vi "Blinking_Led_13.vi"() -> ()   [LabVIEW 2018]
uses:
  <vilib>/MakerHub/LINX/Public/Peripherals/Digital/Digital Write 1 Chan.vi
  <vilib>/MakerHub/LINX/Public/Peripherals/Digital/Digital Write N Chans.vi
  <vilib>/MakerHub/LINX/Private/Local IO/LinxDigitalWrite.vi
  <vilib>/MakerHub/LINX/Public/Utilities/Check Channel.vi
  <vilib>/MakerHub/LINX/Public/Utilities/Open Serial.vi
  <vilib>/MakerHub/LINX/Private/Utilties/Generate Error.vi
  <vilib>/MakerHub/LINX/LMH-LINX.lvlib
panel:
  in  "milliseconds Toff":u32=500
  in  "milliseconds Ton":u32=500
  in  "Repeticiones blink":i32=6
  in  "DO Channel":u8=13 min=2 step=1
  in  "Serial Port":refnum<visa-resource-name>="COM3"
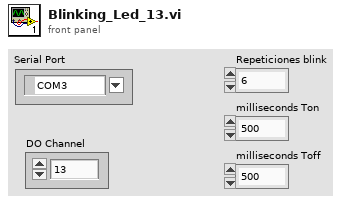
[diagram p1: front panel]
types:
  T1 = typedef "LMH-LINX.lvlib/LINX Ref.ctl" = cluster{"IO":T2, "Interface":T3, "LINX Device Config":T4}
  T2 = typedef "LMH-LINX.lvlib/Platform.ctl" = enum16{"Remote", "Local"}
  T3 = typedef "LMH-LINX.lvlib/Interface.ctl" = enum16{"Serial", "TCP"}
  T4 = typedef "LMH-LINX.lvlib/Device.lvlib/LINX Device Config.ctl" = cluster{"Interface":T3, "COM Port":refnum<visa-resource-name>, "TCP Configuration":T5, "Device Family":u8, "Device ID":u8, "Device Name":string, "TCP Ref":refnum<k5>, "Channels":T6}
  T5 = typedef "LMH-LINX.lvlib/Device.lvlib/TCP Config.ctl" = cluster{"IP Address":string, "Port":u16}
  T6 = typedef "LMH-LINX.lvlib/Channels.ctl" = cluster{"DI":u8[], "DO":u8[], "AI":u8[], "AO":u8[], "PWM":u8[], "QE":u8[], "UART":u8[], "I2C 2":u8[], "SPI":u8[], "CAN":u8[], "Servo":u8[], "AI Ref (V)":dbl, "AI Resolution (Bits)":u8, "AO Ref (V)":dbl, "AO Resolution (Bits)":u8}
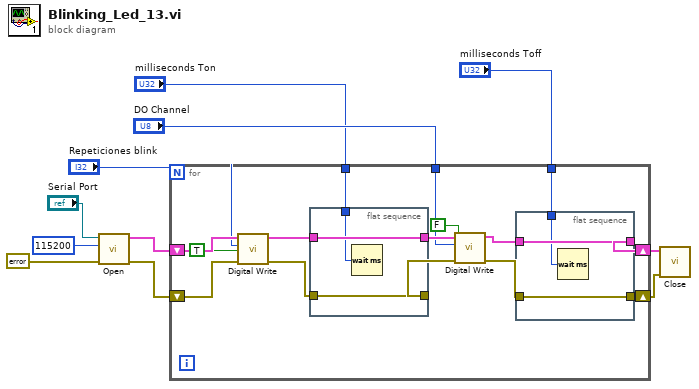
[diagram p0: block diagram]
diagram:
  n1 = call-poly <vilib>:"Open.vi"("Error In"=errorcluster {"status"=FALSE, "code"=0, "source"=""}, "Baud Rate Override"=u32 115200, "Serial Port"="Serial Port") -> ("Error Out"=w7:errorcluster, "LINX Resource"=w8:T1)  [unwired: 6 in, 1 out]
  n2 = for {
    N: "Repeticiones blink" -> [_]
    tunnel: "DO Channel" -> [w14]
    shift-right: [w17] -> w5
    shift-left: w8 -> [w26]
    shift-right: [w21] -> w6
    shift-left: w7 -> [w25]
    tunnel: "milliseconds Ton" -> [w13]
    tunnel: "milliseconds Toff" -> [w12]
    n3 = call-poly <vilib>:"Digital Write.vi"("Error In"=w25, "Output Value"=TRUE, "DO Channel"=w14, "LINX Resource"=w26) -> ("Error Out"=w24:errorcluster, "LINX Resource"=w20:T1)  [unwired: 6 in]
    n4 = flat-sequence {
      tunnel: w24 -> [w32]
      tunnel: [w32] -> w23
      tunnel: [w31] -> w19
      tunnel: w20 -> [w31]
      tunnel: w13 -> [w30]
      frame #0 {
        n5 = Wait (ms)(milliseconds to wait=w30) -> ()  [unwired: 1 out]
      }
    }
    n6 = call-poly <vilib>:"Digital Write.vi"("Error In"=w23, "Output Value"=FALSE, "DO Channel"=w14, "LINX Resource"=w19) -> ("Error Out"=w22:errorcluster, "LINX Resource"=w18:T1)  [unwired: 6 in]
    n7 = flat-sequence {
      tunnel: w22 -> [w29]
      tunnel: [w29] -> w21
      tunnel: [w28] -> w17
      tunnel: w18 -> [w28]
      tunnel: w12 -> [w27]
      frame #0 {
        n8 = Wait (ms)(milliseconds to wait=w27) -> ()  [unwired: 1 out]
      }
    }
  }
  n9 = call <vilib>:"Close.vi"("Error In"=w6, "LINX Resource"=w5) -> ()  [unwired: 9 in, 1 out]
